vi "ExecuteSkill.vi"(0 "object in":refnum<class "KickToSkill_v2.lvclass">, 2 "Robot in":refnum<class "Robot.lvclass">, 4 "GameRef":refnum<data-value>, 5 "error in (no error)":errorcluster) -> (14 "object out":refnum<class "KickToSkill_v2.lvclass">, 16 "Robot out":refnum<class "Robot.lvclass">, 19 "error out":errorcluster)   [LabVIEW 2023, in "KickToSkill_v2.lvclass"]
uses:
  KickToSkill_v2.lvclass
  C:/Users/ebert/Documents/codes/SSL/repo/SSL_AI/GoToSkill_v2_class/GoToSkill_v2.lvclass
  Robot_class/Robot.lvclass
  Game_class/Game.lvclass
  Game_class/Navigation/driveMode.ctl
  KickToSkill_v2.lvclass/KickToSkill_v2.ctl
  Robot_class/Robot.lvclass/Robot.ctl
  Game_class/Game.lvclass/Game.ctl
  Object_class/Object.lvclass/Object.ctl
  Game_class/Read BallRef.vi
  Object_class/Read position(x,y).vi
  Robot_class/Read dest_x_kick.vi
  Robot_class/Read dest_y_kick.vi
  Robot_class/Write kick_x.vi
  Robot_class/Write kick_z.vi
  Ball_class/Ball.lvclass
  C:/Users/ebert/Documents/codes/SSL/repo/SSL_AI/Object_class/Object.lvclass
  GoToSkill_v2_class/GoToSkill_v2.lvclass
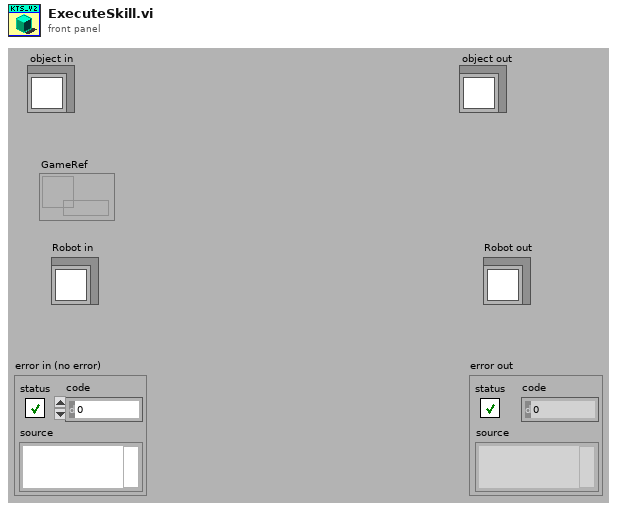
[diagram p1: front panel]
types:
  T1 = typedef "driveMode.ctl" = enum16{"Fast", "SafeDrive"}
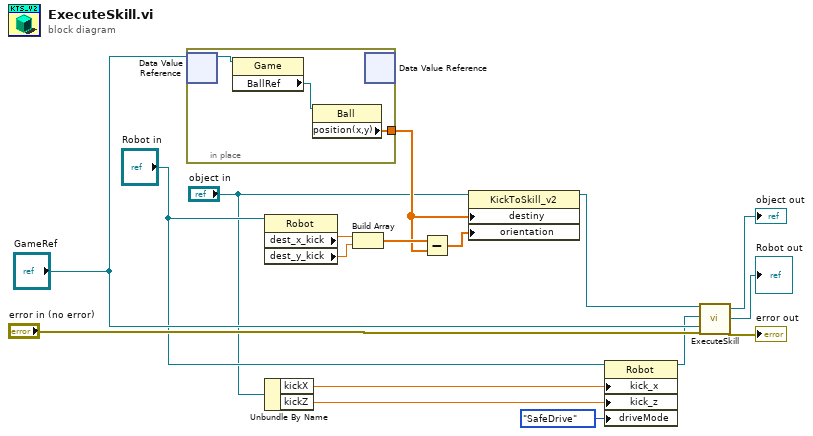
[diagram p0: block diagram]
diagram:
  n1 = in-place {
    in-place-border: [w18] -> w8
    n2 = in-place-dvr #1("GameRef") -> (w20:refnum<class "Game.lvclass">)  [unwired: 1 out]
    n3 = property class="Game"(reference=w20) -> ("BallRef"=w19:refnum<class "Ball.lvclass">)  [unwired: 1 in, 2 out]
    n4 = property class="Ball"(reference=w19) -> ("position(x,y)"=w18:dbl[])  [unwired: 1 in, 2 out]
    n5 = in-place-dvr #1() -> ()  [unwired: 1 in, 2 out]
  }
  n6 = property class="Robot"(reference="Robot in") -> ("dest_x_kick"=w13:dbl, "dest_y_kick"=w12:dbl)  [unwired: 1 in, 2 out]
  n7 = Unbundle By Name("object in") -> ("kickX"=w2:dbl, "kickZ"=w1:dbl)
  n8 = Build Array(w13, w12) -> (w11:dbl[])
  n9 = Subtract(x=w11, y=w8) -> (x-y=w9:dbl[])
  n10 = property class="KickToSkill_v2"(reference="object in", "destiny"=w8, "orientation"=w9) -> (reference out=w7:refnum<class "KickToSkill_v2.lvclass">)  [unwired: 1 in, 1 out]
  n11 = property class="Robot"(reference="Robot in", "kick_x"=w2, "kick_z"=w1, "driveMode"=driveMode."SafeDrive") -> (reference out=w5:refnum<class "Robot.lvclass">)  [unwired: 1 in, 1 out]
  n12 = call-parent "ExecuteSkill.vi"("object in"=w7, "Robot in"=w5, "GameRef"="GameRef", "error in (no error)"="error in (no error)") -> ("object out"=→"object out":refnum<class "KickToSkill_v2.lvclass">, "Robot out"=→"Robot out":refnum<class "Robot.lvclass">, "error out"=→"error out":errorcluster)  [unwired: 13 in]
